vi "Load State Machine.vi"   [LabVIEW 2013]
uses:
  typedefs/singleUseSubstate.ctl
  typedefs/fg_typedef.ctl
  <vilib>/Rock Robotics/WPI/Solenoid/WPI_SolenoidValue.ctl
  typedefs/subStates.ctl
  <vilib>/Rock Robotics/WPI/Solenoid/WPI_SolenoidGetEnum.vi
panel:
  # "A State Machine to Handle Loading for Either High or Low Goal Shots"
types:
  T1 = enum16{"Shooter Solenoid", "Latch Solenoid", "Right Up Sensor", "Right Down Sensor", "Hold Sensor"}
  T2 = typedef "fg_typedef.ctl" = enum16{"Get", "Set"}
  T3 = typedef "singleUseSubstate.ctl" = enum16{"null", "wait", "shift high", "shift low", "cock shooter", "retract shooter", "latch", "unlatch"}
  T4 = typedef "WPI_SolenoidValue.ctl" = enum16{"Off", "On", "Forward", "Reverse"}
  T5 = typedef "subStates.ctl" = enum16{"null", "wait", "driver control", "auto", "manual override", "hold position", "rotate", "pickup", "pass", "load", "goto shoot", "shoot high goal", "shoot low goal", "cancel arm", "cancel shooter", "end"}
  T6 = typedef "WPI_DigitalInputDevRef.ctl" = cluster{"DevStatus":errorcluster, "DIO Channel":T7, "Digital Module":T8}
  T7 = typedef "FPGA_DIOChannel.ctl" = enum8{"DIO 1", "DIO 2", "DIO 3", "DIO 4", "DIO 5", "DIO 6", "DIO 7", "DIO 8", "DIO 9", "DIO 10", "DIO 11", "DIO 12", "DIO 13", "DIO 14", "Invalid"}
  T8 = typedef "FPGA_TypedefDigitalModule.ctl" = enum16{"Digital Module 1", "Digital Module 2"}
  T9 = typedef "WPI_SolenoidDevRef.ctl" = cluster{"DevStatus":errorcluster, "Solenoid Module":T10, "Forward Solenoid Channel":T11, "Reverse Solenoid Channel":T11}
  T10 = typedef "FPGA_TypedefSolenoidModule.ctl" = enum16{"Solenoid Module 1", "Solenoid Module 2"}
  T11 = typedef "WPI_SolenoidChannel.ctl" = enum8{"Solenoid 1", "Solenoid 2", "Solenoid 3", "Solenoid 4", "Solenoid 5", "Solenoid 6", "Solenoid 7", "Solenoid 8", "Invalid"}
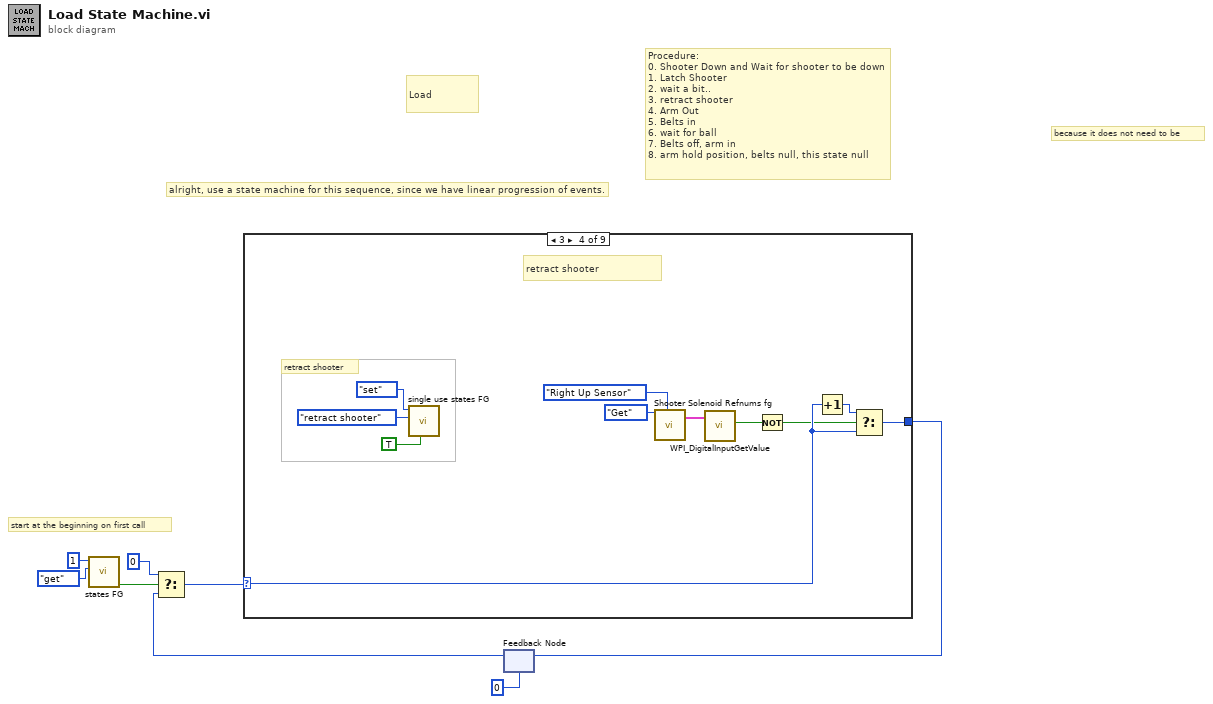
[diagram p0: block diagram]
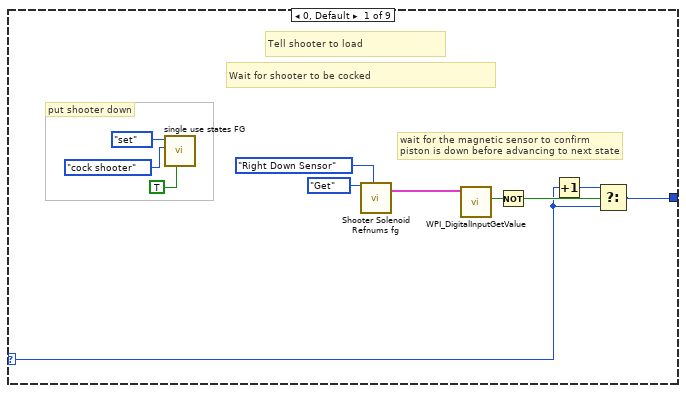
[diagram p2: hidden frame]
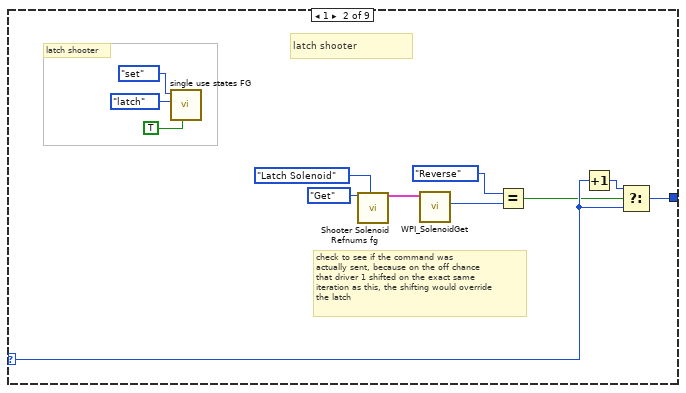
[diagram p3: hidden frame]
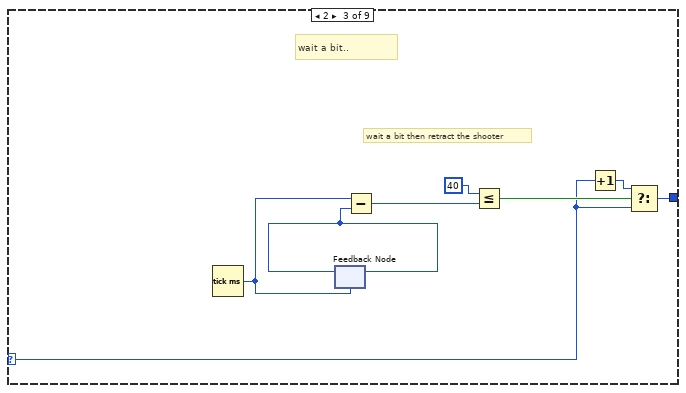
[diagram p4: hidden frame]
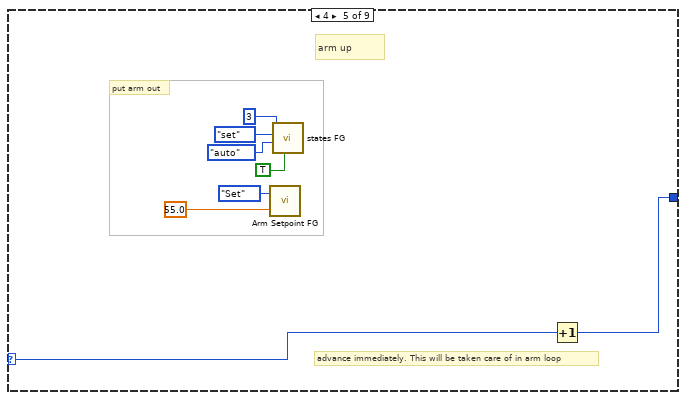
[diagram p5: hidden frame]
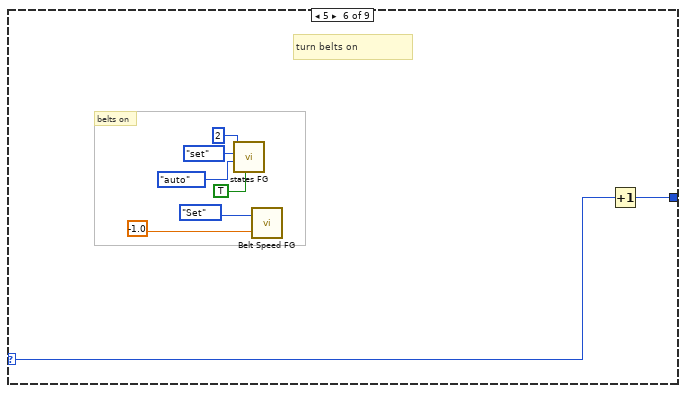
[diagram p6: hidden frame]
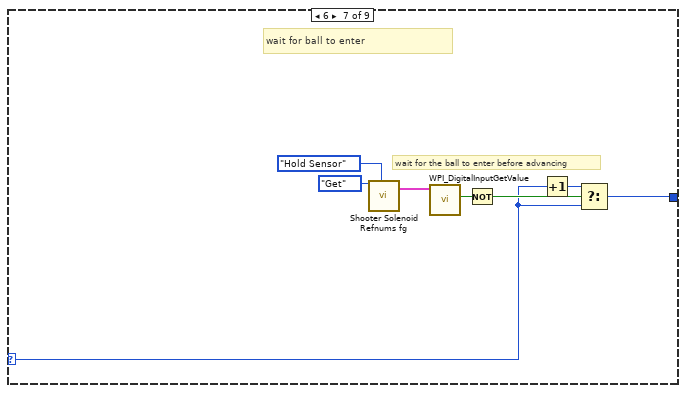
[diagram p7: hidden frame]
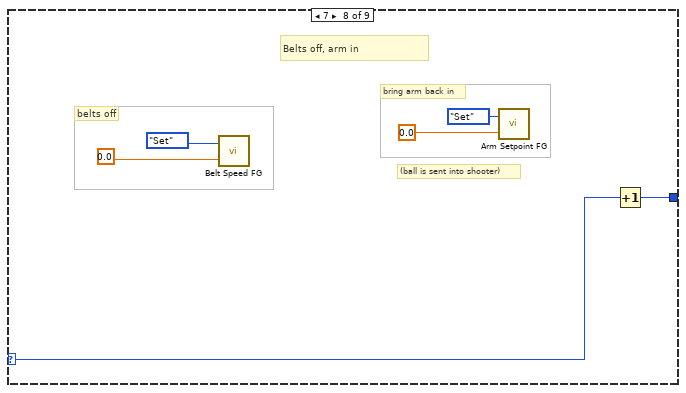
[diagram p8: hidden frame]
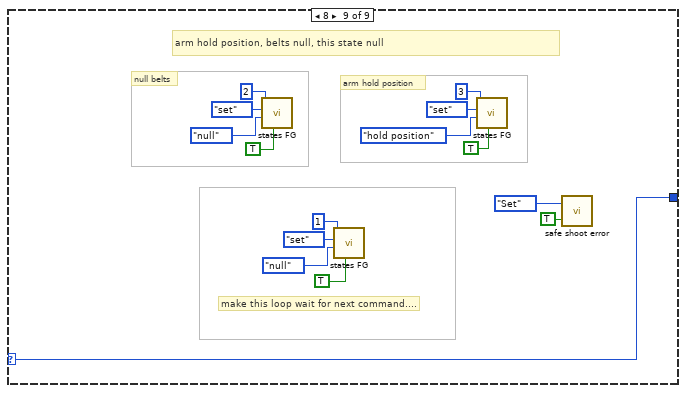
[diagram p9: hidden frame]
diagram:
  # "because it does not need to be"
  # "start at the beginning on first call"
  # "Load"
  # "Procedure: \n0. Shooter Down and Wait for shooter to be down\n1. Latch Shooter\n2. wait a bit..\n3. retract shooter\n4. Arm Out\n5. Belts in\n6. wait for ball\n7. Belts off, arm in\n8. arm hold position, belts null, this state null"
  # "alright, use a state machine for this sequence, since we have linear progression of events."
  n1 = call "states FG.vi"("menu (get)"=enum16{"set", "get"}."get", "Loop ID"=1) -> ("first call?"=w1:bool)  [unwired: 6 in, 3 out]
  n2 = feedback #1(u8 0) -> (w2:u8)
  n3 = Select(t=u8 0, s=w1, f=w2) -> (s? t:f=w4:u8)
  n4 = case shown="3" w4 {
    selector: w4 -> [w12 w27 w33 w44 w53 w61 w71 w76 w86]
    tunnel: [w13 w28 w35 w43 w52 w60 w70 w75 w86] -> w7
    frame 0, Default {
      # "Wait for shooter to be cocked"
      # "wait for the magnetic sensor to confirm \npiston is down before advancing to next state"
      # "Tell shooter to load"
      # "put shooter down"
      n5 = call "single use states FG.vi"("exit in"=TRUE, "substate"=singleUseSubstate."cock shooter", "menu (get)"=enum16{"set", "get"}."set") -> ()  [unwired: 5 in, 4 out]
      n6 = call "Shooter Solenoid Refnums fg.vi"("Menu"=fg_typedef."Get", "DevRef to Get"=T1."Right Down Sensor") -> ("Selected Sensor"=w9:T6)  [unwired: 15 in, 2 out]
      n7 = call <vilib>:"WPI_DigitalInputGetValue.vi"("DigitalInputDevRef"=w9) -> ("Value"=w16:bool)  [unwired: 8 in, 2 out]
      n8 = Not(x=w16) -> (.not. x?=w14:bool)
      n9 = Increment(x=w12) -> (x+1=w15:u8)
      n10 = Select(t=w15, s=w14, f=w12) -> (s? t:f=w13:u8)
    }
    frame 1 {
      # "latch shooter"
      # "check to see if the command was\nactually sent, because on the off chance\nthat driver 1 shifted on the exact same\niteration as this, the shifting would override\nthe latch"
      # "latch shooter"
      n11 = call "single use states FG.vi"("exit in"=TRUE, "substate"=singleUseSubstate."latch", "menu (get)"=enum16{"set", "get"}."set") -> ()  [unwired: 5 in, 4 out]
      n12 = call "Shooter Solenoid Refnums fg.vi"("Menu"=fg_typedef."Get", "DevRef to Get"=T1."Latch Solenoid") -> ("Selected Solenoid"=w23:T9)  [unwired: 15 in, 2 out]
      n13 = call-poly <vilib>:"WPI_SolenoidGet.vi"("SolenoidDevRef"=w23) -> ("Value"=w22:T4)  [unwired: 8 in, 2 out]
      n14 = Equal?(x=WPI_SolenoidValue."Reverse" ("Value"), y=w22) -> (x = y?=w20:bool)
      n15 = Increment(x=w27) -> (x+1=w26:u8)
      n16 = Select(t=w26, s=w20, f=w27) -> (s? t:f=w28:u8)
    }
    frame 2 {
      # "wait a bit.."
      # "wait a bit then retract the shooter"
      n17 = Tick Count (ms)() -> (millisecond timer value=w37:u32)
      n18 = feedback #2(w37) -> (w38:u32)
      n19 = feedback-in #2(w38) -> ()
      n20 = Subtract(x=w37, y=w38) -> (x-y=w36:u32)
      n21 = Less Or Equal?(x=u32 40, y=w36) -> (x <= y?=w34:bool)
      n22 = Increment(x=w33) -> (x+1=w32:u8)
      n23 = Select(t=w32, s=w34, f=w33) -> (s? t:f=w35:u8)
    }
    frame 3 {
      # "retract shooter"
      # "retract shooter"
      n24 = call "single use states FG.vi"("exit in"=TRUE, "substate"=singleUseSubstate."retract shooter", "menu (get)"=enum16{"set", "get"}."set") -> ()  [unwired: 5 in, 4 out]
      n25 = call "Shooter Solenoid Refnums fg.vi"("Menu"=fg_typedef."Get", "DevRef to Get"=T1."Right Up Sensor") -> ("Selected Sensor"=w42:T6)  [unwired: 15 in, 2 out]
      n26 = call <vilib>:"WPI_DigitalInputGetValue.vi"("DigitalInputDevRef"=w42) -> ("Value"=w41:bool)  [unwired: 8 in, 2 out]
      n27 = Not(x=w41) -> (.not. x?=w40:bool)
      n28 = Increment(x=w44) -> (x+1=w47:u8)
      n29 = Select(t=w47, s=w40, f=w44) -> (s? t:f=w43:u8)
    }
    frame 4 {
      # "arm up"
      # "advance immediately. This will be taken care of in arm loop"
      # "put arm out"
      n30 = call "Arm Setpoint FG.vi"("Setpoint In"=55.0, "Menu"=fg_typedef."Set") -> ()  [unwired: 1 out]
      n31 = call "states FG.vi"("exit in"=TRUE, "subState in"=subStates."auto", "menu (get)"=enum16{"set", "get"}."set", "Loop ID"=3) -> ()  [unwired: 4 in, 4 out]
      n32 = Increment(x=w53) -> (x+1=w52:u8)
    }
    frame 5 {
      # "belts on"
      # "turn belts on"
      n33 = call "states FG.vi"("exit in"=TRUE, "subState in"=subStates."auto", "menu (get)"=enum16{"set", "get"}."set", "Loop ID"=2) -> ()  [unwired: 4 in, 4 out]
      n34 = call "Belt Speed FG.vi"("Speed In"=-1.0 ("Setpoint In"), "Menu"=fg_typedef."Set") -> ()  [unwired: 1 out]
      n35 = Increment(x=w61) -> (x+1=w60:u8)
    }
    frame 6 {
      # "wait for the ball to enter before advancing"
      # "wait for ball to enter"
      n36 = call "Shooter Solenoid Refnums fg.vi"("Menu"=fg_typedef."Get", "DevRef to Get"=T1."Hold Sensor") -> ("Selected Sensor"=w67:T6)  [unwired: 15 in, 2 out]
      n37 = call <vilib>:"WPI_DigitalInputGetValue.vi"("DigitalInputDevRef"=w67) -> ("Value"=w73:bool)  [unwired: 8 in, 2 out]
      n38 = Not(x=w73) -> (.not. x?=w72:bool)
      n39 = Increment(x=w71) -> (x+1=w74:u8)
      n40 = Select(t=w74, s=w72, f=w71) -> (s? t:f=w70:u8)
    }
    frame 7 {
      # "bring arm back in"
      # "Belts off, arm in"
      # "(ball is sent into shooter)"
      # "belts off"
      n41 = call "Belt Speed FG.vi"("Speed In"=0.0 ("Setpoint In"), "Menu"=fg_typedef."Set") -> ()  [unwired: 1 out]
      n42 = call "Arm Setpoint FG.vi"("Setpoint In"=0.0, "Menu"=fg_typedef."Set") -> ()  [unwired: 1 out]
      n43 = Increment(x=w76) -> (x+1=w75:u8)
    }
    frame 8 {
      # "arm hold position, belts null, this state null"
      # "make this loop wait for next command...."
      # "arm hold position"
      # "null belts"
      n44 = call "states FG.vi"("exit in"=TRUE, "subState in"=subStates."null", "menu (get)"=enum16{"set", "get"}."set", "Loop ID"=2) -> ()  [unwired: 4 in, 4 out]
      n45 = call "states FG.vi"("exit in"=TRUE, "subState in"=subStates."null", "menu (get)"=enum16{"set", "get"}."set", "Loop ID"=1) -> ()  [unwired: 4 in, 4 out]
      n46 = call "states FG.vi"("exit in"=TRUE, "subState in"=subStates."hold position", "menu (get)"=enum16{"set", "get"}."set", "Loop ID"=3) -> ()  [unwired: 4 in, 4 out]
      n47 = call "safe shoot error.vi"("Can Shoot Safely?"=TRUE, "Menu"=fg_typedef."Set") -> ()  [unwired: 1 out]
    }
  }
  n48 = feedback-in #1(w7) -> ()
